vi "Change Password.vi"(8 "error in (no error)":errorcluster, 11 "Configuration in":refnum<class "Configuration.lvclass">) -> (0 "error out":errorcluster, 3 "Configuration out":refnum<class "Configuration.lvclass">)   [LabVIEW 2016, in "Configuration.lvlib" / "Configuration.lvclass"]
uses:
  <userlib>/Configuration Dialog Actor/Configuration.lvclass
  C:/Program Files (x86)/National Instruments/LabVIEW 2016/vi.lib/ActorFramework/Actor/Actor.lvclass
  <vilib>/ActorFramework/Actor/Actor.lvclass/Actor.ctl
  <userlib>/Configuration Dialog Actor/Configuration.lvclass/Configuration.ctl
  <userlib>/Common Components/Function Messages/Log in MsgList Msg/Log in MsgList Msg.lvclass/Log in MsgList Msg.ctl
  <vilib>/ActorFramework/Message Enqueuer/Message Enqueuer.lvclass/Message Enqueuer.ctl
  <vilib>/ActorFramework/Message Enqueuer/Enqueue.vi
  <userlib>/Common Components/Function Messages/Log in MsgList Msg/Log in MsgList Msg.lvclass
  C:/Program Files (x86)/National Instruments/LabVIEW 2016/vi.lib/ActorFramework/Message/Message.lvclass
  <vilib>/ActorFramework/Message Priority Queue/Priority Enqueue.vi
  <userlib>/_OpenG.lib/md5/md5.llb/MD5 Message Digest (Hexadecimal String)__ogtk.vi
  <vilib>/ActorFramework/Actor/Actor.lvclass
  <vilib>/Utility/config.llb/NI_LVConfig.lvlib
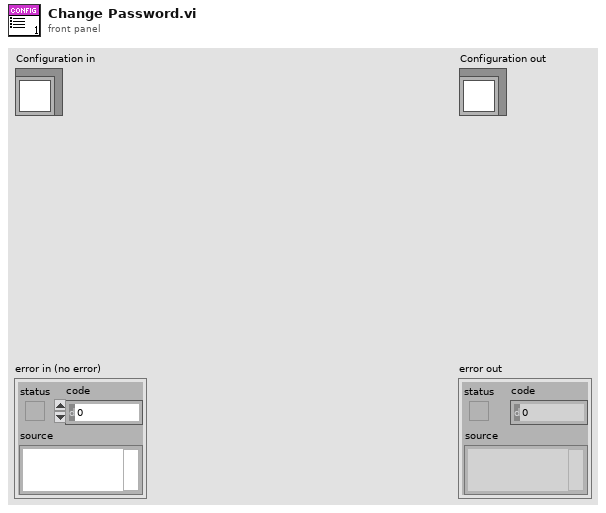
[diagram p1: front panel]
types:
  T1 = typedef "NI_LVConfig.lvlib/Config Data RefNum.ctl" = refnum<k1>
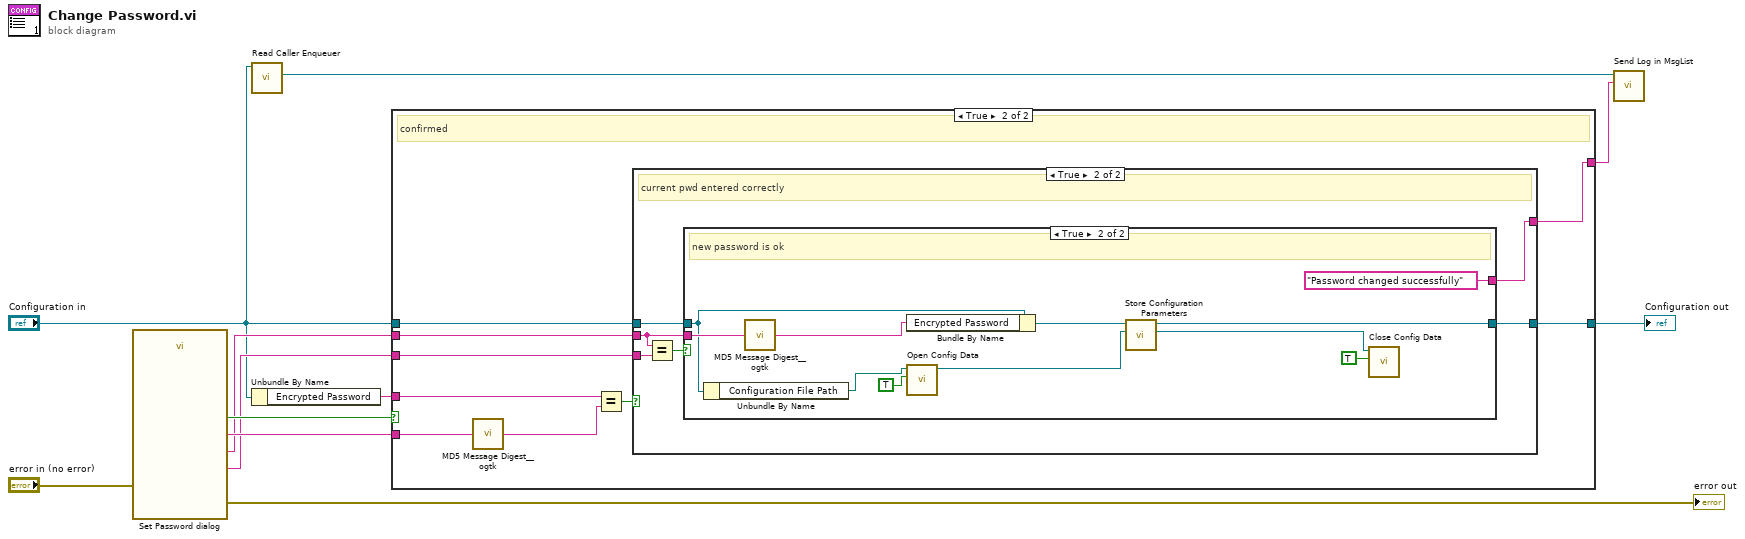
[diagram p0: block diagram]
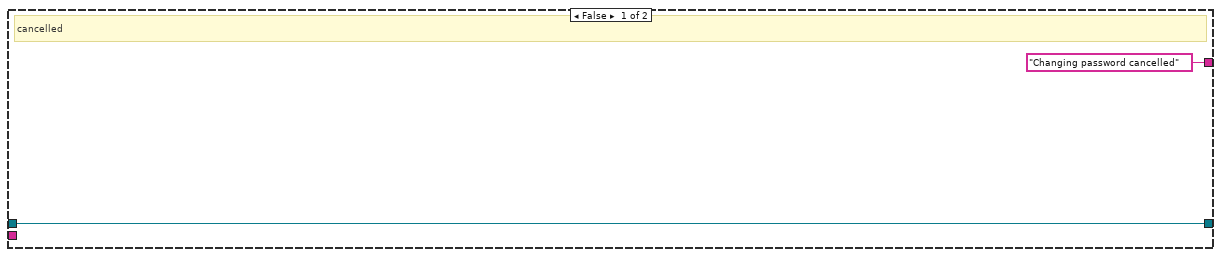
[diagram p2: hidden frame]
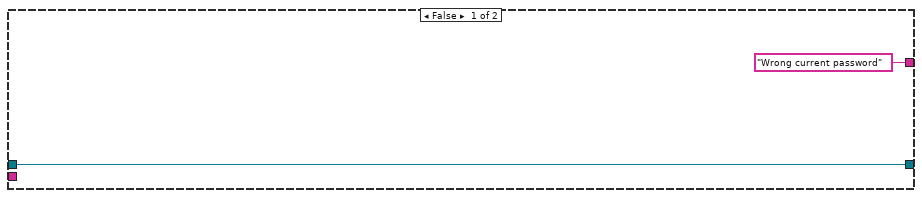
[diagram p3: hidden frame]
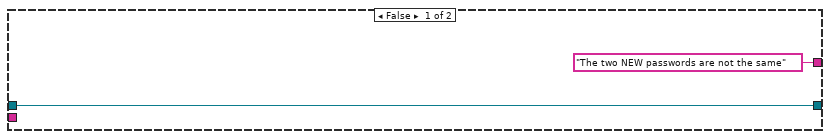
[diagram p4: hidden frame]
diagram:
  n1 = call <userlib>:"Set Password dialog.vi"("error in (no error)"="error in (no error)") -> ("Please re-enter the New password again"=w7:string, "Please enter the NEW password"=w8:string, "Please enter the current password"=w10:string, "Confirm"=w11:bool, "error out"=→"error out":errorcluster)  [unwired: 14 in]
  n2 = call <vilib>:"Read Caller Enqueuer.vi"("Actor"="Configuration in") -> ("Caller Enqueuer"=w4:refnum<class "Message Enqueuer.lvclass">)  [unwired: 10 in]
  n3 = Unbundle By Name("Configuration in") -> ("Encrypted Password"=w9:string)
  n4 = case shown="True" w11 {
    tunnel: w10 -> [_ w22]
    tunnel: w9 -> [_ w21]
    tunnel: w8 -> [_ w19]
    tunnel: w7 -> [_ w15]
    tunnel: "Configuration in" -> [w13 w18]
    tunnel: [w13 w17] -> w6
    tunnel: ["Changing password cancelled" ("Msg") w14] -> w3
    frame False {
      # "cancelled"
    }
    frame True {
      # "confirmed"
      n5 = call-poly <userlib>:"MD5 Message Digest__ogtk.vi"("Message"=w22) -> ("MD5 Message Digest"=w20:string)
      n6 = Equal?(x=w21, y=w20) -> (x = y?=w16:bool)
      n7 = case shown="True" w16 {
        tunnel: w19 -> [_ w28]
        tunnel: w18 -> [w24 w30]
        tunnel: [w24 w29] -> w17
        tunnel: w15 -> [_ w27]
        tunnel: ["Wrong current password" w25] -> w14
        frame False {
        }
        frame True {
          # "current pwd entered correctly"
          n8 = Equal?(x=w28, y=w27) -> (x = y?=w26:bool)
          n9 = case shown="True" w26 {
            tunnel: w28 -> [_ w43]
            tunnel: w30 -> [w31 w37]
            tunnel: [w31 w35] -> w29
            tunnel: ["The two NEW passwords are not the same" "Password changed successfully"] -> w25
            frame False {
            }
            frame True {
              # "new password is ok"
              n10 = Unbundle By Name(w37) -> ("Configuration File Path"=w38:path)
              n11 = call-poly <userlib>:"MD5 Message Digest__ogtk.vi"("Message"=w43) -> ("MD5 Message Digest"=w42:string)
              n12 = Bundle By Name(cluster=w37, "Encrypted Password"=w42) -> (w36:refnum<class "Configuration.lvclass">)
              n13 = call <vilib>:"Open Config Data.vi"("create file if necessary (T)"=TRUE, "configuration file path"=w38) -> ("refnum"=w34:T1)  [unwired: 7 in, 2 out]
              n14 = call-dynamic "Store Configuration Parameters.vi"("refnum"=w34, "Configuration in"=w36) -> ("refnum out"=w33:T1, "Configuration out"=w35:refnum<class "Configuration.lvclass">)  [unwired: 7 in, 1 out]
              n15 = call <vilib>:"Close Config Data.vi"("write file if changed (T)"=TRUE, "refnum"=w33) -> ()  [unwired: 8 in, 2 out]
            }
          }
        }
      }
    }
  }
  "Configuration out" <- w6
  n16 = call <userlib>:"Send Log in MsgList.vi"("Msg"=w3, "Message Enqueuer"=w4) -> ()  [unwired: 8 in, 2 out]
